vi "flushTelQueue.vi"(8 "error in (no error)":errorcluster, 10 "queueName":enum16{"queueFromDds", "queueToDds"}(ring), 11 "TcpServer in":refnum<class "TcpServer.lvclass">) -> (0 "error out":errorcluster, 2 "telemetry flushed":string[](array[string]), 3 "TcpServer out":refnum<class "TcpServer.lvclass">)   [LabVIEW 2018, in "TcpServer.lvclass"]
doc: "Flush the queue with telemetry. Use the queueName enum control to select either queueFromDds or queueToDds."
uses:
  TcpServer.lvclass
  TcpServer.lvclass/TcpServer.ctl
  TcpServerTel/TcpServerTel.lvclass
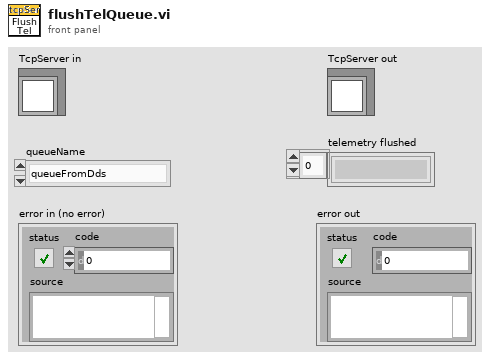
[diagram p1: front panel]
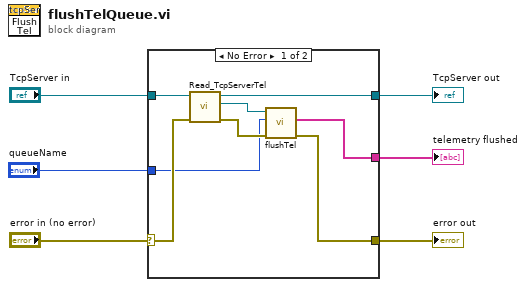
[diagram p0: block diagram]
diagram:
  n1 = case shown="No Error" "error in (no error)" {
    selector: "error in (no error)" -> [w14 w15]
    tunnel: [w11 w15] -> w6
    tunnel: "TcpServer in" -> [w13 w16]
    tunnel: [w9 w16] -> w3
    tunnel: [w8 _] -> w2
    tunnel: "queueName" -> [w7 _]
    frame No Error {
      n2 = call "Read_TcpServerTel.vi"("error in (no error)"=w14, "TcpServer in"=w13) -> ("error out"=w12:errorcluster, "TcpServerTel.lvclass"=w10:refnum<class "TcpServerTel.lvclass">, "TcpServer out"=w9:refnum<class "TcpServer.lvclass">)  [unwired: 7 in]
      n3 = call "flushTel.vi"("error in (no error)"=w12, "queueName"=w7, "tcpServerTel in"=w10) -> ("error out"=w11:errorcluster, "telemetry flushed"=w8:string[])  [unwired: 6 in, 1 out]
    }
    frame Error {
    }
  }
  "error out" <- w6
  "TcpServer out" <- w3
  "telemetry flushed" <- w2
